vi "4145 Graphics Plot.vi"(0 "4145_GPIB_COM_IN":T3={"Address_string"="17", "timeout ms"=25000, "Terminator"=",", "LoggerQueue"=refnum}, 1 "4145_X_Axis_IN":T6={"X axis"=TRUE, "X channel name"="V3", "X scale"=TRUE, "X min"=0.0, "X max"=1.0, "Is X axis VAR 1?"=FALSE} {"X max" format="%^.3e"; "X min" format="%^.3e"}, 2 "4145_Y_Axis_IN":T5={"Y1 channel name"="I3", "Y1 scale"=TRUE, "Y1 min"=0.0, "Y1 max"=0.01} {"Y1 max" format="%^.3e"; "Y1 min" format="%^.3e"}, 3 "4145_Y2_Axis_IN":T4={"Y2 axis"=FALSE, "Y2 channel name"="", "Y2 scale"=TRUE, "Y2 min"=0.0, "Y2 max"=0.01, "# of steps for VAR 2"=0} {"Y2 max" format="%^.3e"; "Y2 min" format="%^.3e"}, 5 "error in":T7) -> (14 "Spreadsheet data":T1, 16 "Spreadsheet formatted":dbl[][](array[numeric]), 19 "error out":T7)   [LabVIEW 2014]
doc: "This VI configures the intrument for graphics display, takes a measurement, waits for a Service Request, then reads the appropriate data, converts the data into plottable form, and plots the configured graph. The graph must be scaled by hand (limitation of Labview 2.5) to make it look identical to the graph on the instrument."
uses:
  typedef/4145_X_Axis.ctl
  typedef/4145_Y_Axis.ctl
  typedef/4145_Y2_Axis.ctl
  typedef/4145_GPIB_Com.ctl
  typedef/4145_que_msg.ctl
  typedef/4145 command enum.ctl
  typedef/4145 Spreadsheet data.ctl
  <vilib>/Utility/miscctls.llb/LVRangeTypeDef.ctl
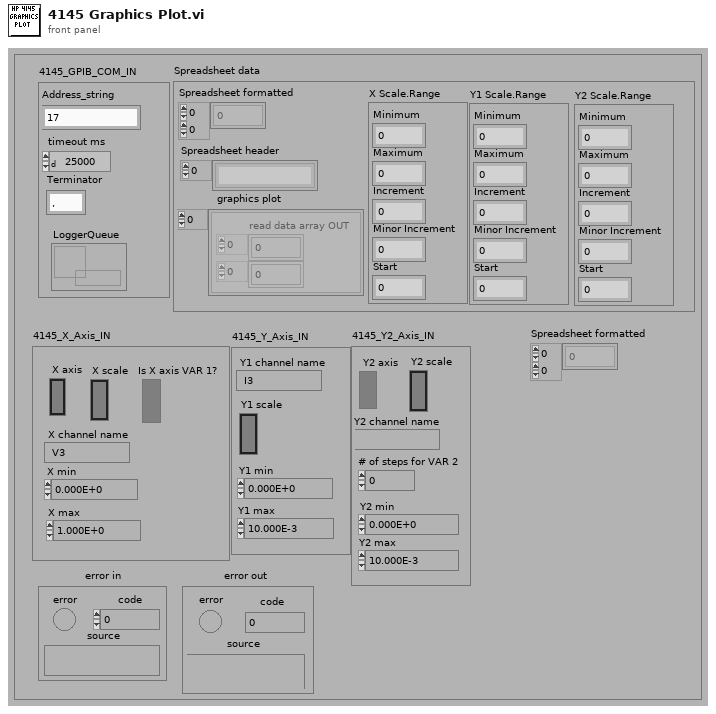
[diagram p1: front panel]
types:
  T1 = typedef "4145 Spreadsheet data.ctl" = cluster{"Spreadsheet formatted":dbl[][], "Spreadsheet header":string[], "graphics plot":cluster{"read data array OUT":dbl[], dbl[]}[], "X Scale.Range":T2, "Y1 Scale.Range ":T2, "Y2 Scale.Range":T2}
  T2 = typedef "LVRangeTypeDef.ctl" = cluster{"Minimum":dbl, "Maximum":dbl, "Increment":dbl, "Minor Increment":dbl, "Start":dbl}
  T3 = typedef "4145_GPIB_Com.ctl" = cluster{"Address_string":string, "timeout ms":u32, "Terminator":string, "LoggerQueue":refnum<queue>}
  T4 = typedef "4145_Y2_Axis.ctl" = cluster{"Y2 axis":bool, "Y2 channel name":string, "Y2 scale":bool, "Y2 min":dbl, "Y2 max":dbl, "# of steps for VAR 2":u16}
  T5 = typedef "4145_Y_Axis.ctl" = cluster{"Y1 channel name":string, "Y1 scale":bool, "Y1 min":dbl, "Y1 max":dbl}
  T6 = typedef "4145_X_Axis.ctl" = cluster{"X axis":bool, "X channel name":string, "X scale":bool, "X min":dbl, "X max":dbl, "Is X axis VAR 1?":bool}
  T7 = cluster{"error":bool, "code":i32, "source":string}
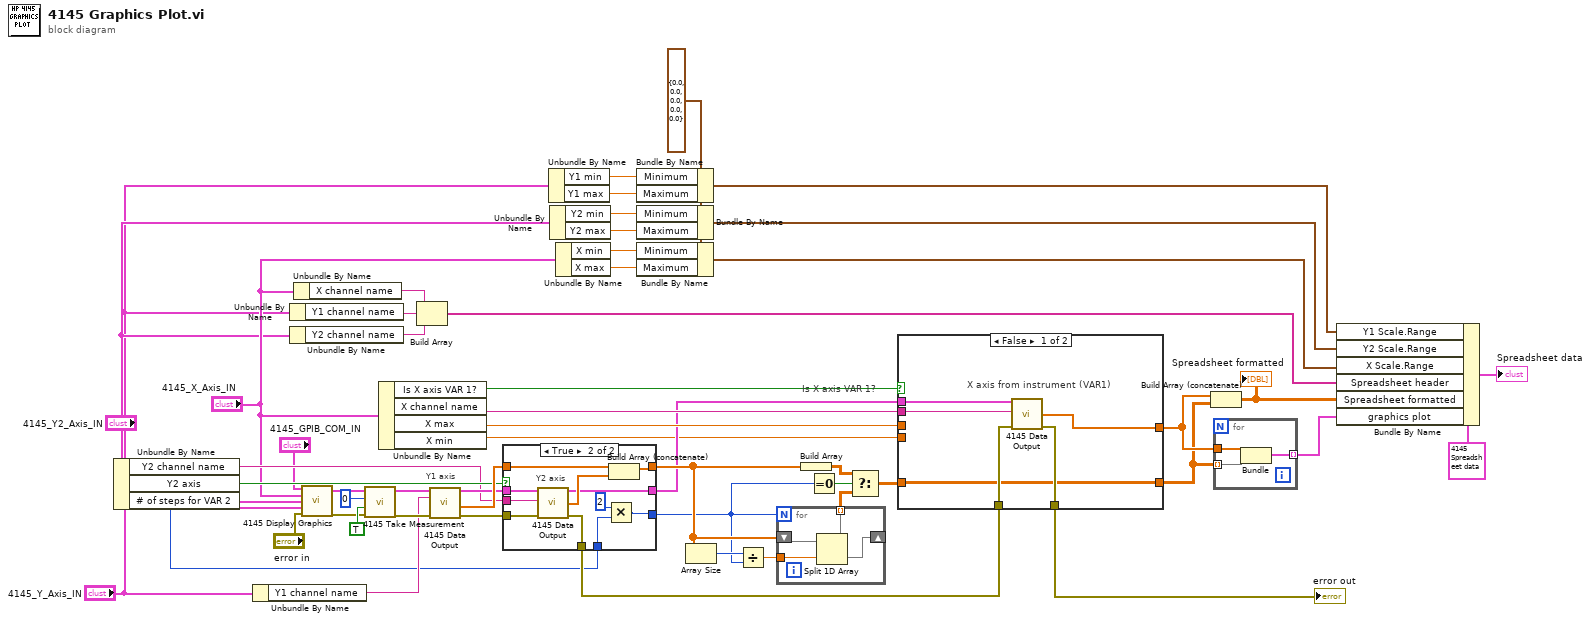
[diagram p0: block diagram]
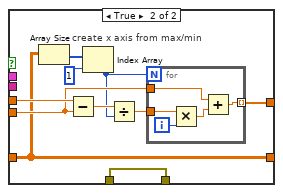
[diagram p3: hidden frame]
diagram:
  w10 = T2 {"Minimum"=0.0, "Maximum"=0.0, "Increment"=0.0, "Minor Increment"=0.0, "Start"=0.0} ("X Scale.Range")
  # "Y1 axis"
  # "Is X axis VAR 1?"
  n1 = Unbundle By Name("4145_Y2_Axis_IN") -> ("Y2 channel name"=w25:string, "Y2 axis"=w27:bool, "# of steps for VAR 2"=w26:u16)
  n2 = Unbundle By Name("4145_Y_Axis_IN") -> ("Y1 channel name"=w33:string)
  n3 = Unbundle By Name("4145_Y_Axis_IN") -> ("Y1 channel name"=w14:string)
  n4 = Unbundle By Name("4145_Y2_Axis_IN") -> ("Y2 channel name"=w17:string)
  n5 = Unbundle By Name("4145_X_Axis_IN") -> ("X channel name"=w18:string)
  n6 = call "4145 Display Graphics.vi"("4145_GPIB_COM_IN"="4145_GPIB_COM_IN", "4145_X_Axis_IN"="4145_X_Axis_IN", "4145_Y2_Axis_IN"="4145_Y2_Axis_IN", "4145_Y_Axis_IN"="4145_Y_Axis_IN", "error in"="error in") -> ("4145_GPIB_COM_OUT"=w31:T3, "error out"=w35:T7)  [unwired: 9 in]
  n7 = call "4145 Take Measurement.vi"("error in"=w35, "wait for SRQ?"=TRUE, "measurement command (single:0)"=u16 0, "4145_GPIB_COM_in"=w31) -> ("error out"=w42:T7, "4145_GPIB_COM_out"=w32:T3)  [unwired: 6 in]
  n8 = Unbundle By Name("4145_X_Axis_IN") -> ("Is X axis VAR 1?"=w36:bool, "X channel name"=w37:string, "X max"=w38:dbl, "X min"=w28:dbl)
  n9 = Build Array(w18, w14, w17) -> (w16:string[])
  n10 = call "4145 Data Output.vi"("4145_GPIB_Param"=w32, "name"=w33, "error in"=w42) -> ("4145_GPIB_COM_OUT"=w30:T3, "read data array OUT"=w44:dbl[], "error out"=w43:T7)  [unwired: 9 in, 1 out]
  n11 = case shown="True" w27 {
    tunnel: w43 -> [w56 w68]
    tunnel: w44 -> [w57 w67]
    tunnel: [w57 w65] -> w48
    tunnel: w25 -> [_ w60]
    tunnel: w26 -> [w54 w63]
    tunnel: [w54 w62] -> w47
    tunnel: [w56 w61] -> w40
    tunnel: w30 -> [w55 w59]
    tunnel: [w55 w58] -> w29
    frame False {
    }
    frame True {
      # "Y2 axis"
      n12 = call "4145 Data Output.vi"("4145_GPIB_Param"=w59, "name"=w60, "error in"=w68) -> ("4145_GPIB_COM_OUT"=w58:T3, "read data array OUT"=w66:dbl[], "error out"=w61:T7)  [unwired: 9 in, 1 out]
      n13 = Multiply(x=2, y=w63) -> (x*y=w62:i32)
      n14 = Build Array (concatenate)(w67, w66) -> (w65:dbl[])
    }
  }
  n15 = Unbundle By Name("4145_Y_Axis_IN") -> ("Y1 min"=w9:dbl, "Y1 max"=w8:dbl)
  n16 = Unbundle By Name("4145_Y2_Axis_IN") -> ("Y2 min"=w7:dbl, "Y2 max"=w6:dbl)
  n17 = Unbundle By Name("4145_X_Axis_IN") -> ("X min"=w5:dbl, "X max"=w4:dbl)
  n18 = Bundle By Name(cluster=w10, "Minimum"=w9, "Maximum"=w8) -> (w1:T2)
  n19 = Bundle By Name(cluster=w10, "Minimum"=w7, "Maximum"=w6) -> (w2:T2)
  n20 = Bundle By Name(cluster=w10, "Minimum"=w5, "Maximum"=w4) -> (w3:T2)
  n21 = Array Size(array=w48) -> (size(s)=w51:i32)
  n22 = Divide(x=w51, y=w47) -> (x/y=w49:dbl)
  n23 = for {
    N: w47 -> [_]
    shift-right: [w71] -> _
    shift-left: w48 -> [w72]
    tunnel: w49 -> [w70]
    tunnel: [w69] -> w50 mode=indexing
    n24 = Split 1D Array(array=w72, index=w70) -> (first subarray=w69:dbl[], second subarray=w71:dbl[])
  }
  n25 = Build Array(w48) -> (w46:dbl[][])
  n26 = Equal To 0?(x=w47) -> (x = 0?=w45:bool)
  n27 = Select(t=w46, s=w45, f=w50) -> (s? t:f=w39:dbl[][])
  n28 = case shown="False" w36 {
    tunnel: w37 -> [w78 _]
    tunnel: w28 -> [_ w85]
    tunnel: w38 -> [_ w88]
    tunnel: [w77 w84] -> w24
    tunnel: w39 -> [w74 w79]
    tunnel: [w76 w80] -> w41
    tunnel: w40 -> [w75 w80]
    tunnel: [w74 w79] -> w23
    tunnel: w29 -> [w73 _]
    frame False {
      # "X axis from instrument (VAR1)"
      n29 = call "4145 Data Output.vi"("4145_GPIB_Param"=w73, "name"=w78, "error in"=w75) -> ("read data array OUT"=w77:dbl[], "error out"=w76:T7)  [unwired: 9 in, 2 out]
    }
    frame True {
      # "create x axis from max/min"
      n30 = Array Size(array=w79) -> (size(s)=w81:i32[])
      n31 = Subtract(x=w88, y=w85) -> (x-y=w87:dbl)
      n32 = Index Array(array=w81, index=1) -> (element=w82:i32)
      n33 = Divide(x=w87, y=w82) -> (x/y=w86:dbl)
      n34 = for {
        N: w82 -> [_]
        tunnel: w86 -> [w92]
        tunnel: w85 -> [w90]
        tunnel: [w89] -> w84 mode=indexing
        i -> [w93]
        n35 = Multiply(x=w92, y=w93) -> (x*y=w91:dbl)
        n36 = Add(x=w90, y=w91) -> (x+y=w89:dbl)
      }
    }
  }
  "error out" <- w41
  n37 = Build Array (concatenate)(w24, w23) -> (w22:dbl[][])
  "Spreadsheet formatted" <- w22
  n38 = for {
    tunnel: w24 -> [w95]
    tunnel: w23 -> [w96] mode=indexing
    tunnel: [w94] -> w15 mode=indexing
    n39 = Bundle("read data array OUT"=w95, w96) -> (w94:cluster{"read data array OUT":dbl[], dbl[]})  [unwired: 1 in]
  }
  n40 = Bundle By Name(cluster=T1 {"Spreadsheet formatted"=[], "Spreadsheet header"=[], "graphics plot"=[], "X Scale.Range"={"Minimum"=0.0, "Maximum"=0.0, "Increment"=0.0, "Minor Increment"=0.0, "Start"=0.0}, "Y1 Scale.Range "={"Minimum"=0.0, "Maximum"=0.0, "Increment"=0.0, "Minor Increment"=0.0, "Start"=0.0}, "Y2 Scale.Range"={"Minimum"=0.0, "Maximum"=0.0, "Increment"=0.0, "Minor Increment"=0.0, "Start"=0.0}} ("Spreadsheet data"), "Y1 Scale.Range"=w1, "Y2 Scale.Range"=w2, "X Scale.Range"=w3, "Spreadsheet header"=w16, "Spreadsheet formatted"=w22, "graphics plot"=w15) -> (→"Spreadsheet data":T1)
